vi "RTS Get Tech Name.vi"(8 "Error In":errorcluster, 10 "Station Owner Names Input":string[](array[string]), 11 "Setup Info":string) -> (0 "Error Out":errorcluster, 2 "Station Owner Names Output":string[](array[string]), 3 "Tech Name":string)   [LabVIEW 2020]
uses:
  Type Definitions/RTS Room Selector.ctl
  <vilib>/Utility/error.llb/whitespace.ctl
panel:
  in  "Tree Selection":T1="Select Room/Stall"
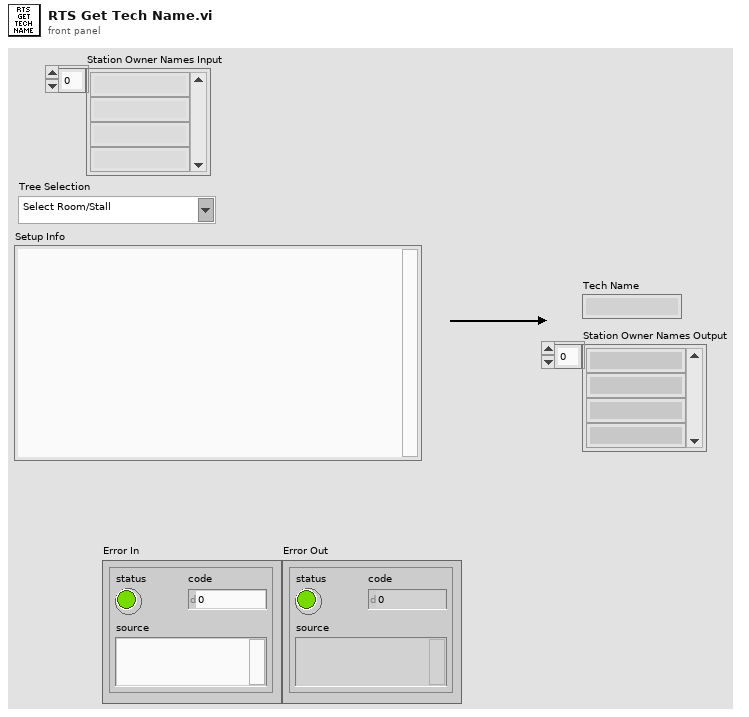
[diagram p1: front panel]
types:
  T1 = typedef "RTS Room Selector.ctl" = string
  T2 = typedef "whitespace.ctl" = u16
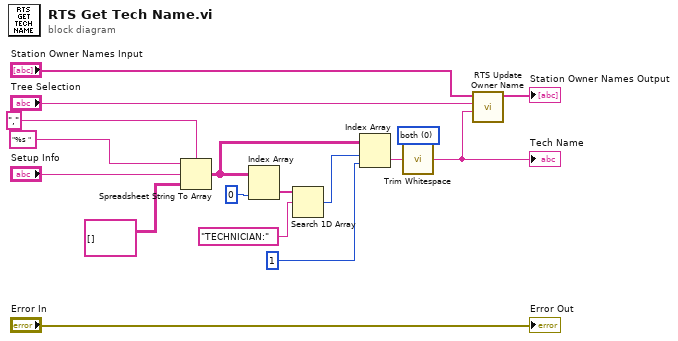
[diagram p0: block diagram]
diagram:
  w6 = T2 0 items=["both", "start of string", "end of string"] ("location (both)")
  n1 = Spreadsheet String To Array(delimiter (Tab)=",", format string="%s ", spreadsheet string="Setup Info", array type (2D Dbl)=string[][] []) -> (array=w10:string[][])
  n2 = Index Array(array=w10, index (col)=0 ("disabled index (col)")) -> (element=w12:string[])  [unwired: 1 in]
  n3 = Search 1D Array(1D array=w12, element="TECHNICIAN:") -> (index of element=w9:i32)  [unwired: 1 in]
  n4 = Index Array(array=w10, index (row)=w9, index (col)=1 ("disabled index (col)")) -> (element=w7:string)
  n5 = call <vilib>:"Trim Whitespace.vi"("string"=w7, "location (both)"=w6) -> ("trimmed string"=w2:string)
  "Tech Name" <- w2
  n6 = call "RTS Update Owner Name.vi"("Insert Value"=w2, "Tree Selection"="Tree Selection", "Station Owner Names Input"="Station Owner Names Input") -> ("Station Owner Names Output"=→"Station Owner Names Output":string[])  [unwired: 7 in, 1 out]
  "Error Out" <- "Error In"
